vi "Copy Channel Properties.vi"(6 "Base Channel":string, 8 "error in (no error)":errorcluster, 9 "New Channel in":string, 10 "Group Name in":string, 11 "TDMS Log File in":refnum<class "TDMS Log File.lvclass">) -> (0 "error out":errorcluster, 1 "New Channel out":string, 2 "Group Name out":string, 3 "TDMS Log File out":refnum<class "TDMS Log File.lvclass">)   [LabVIEW 2015, in "TDMS Log File.lvclass"]
uses:
  TDMS Log File.lvclass
  TDMS Log File.lvclass/TDMS Log File.ctl
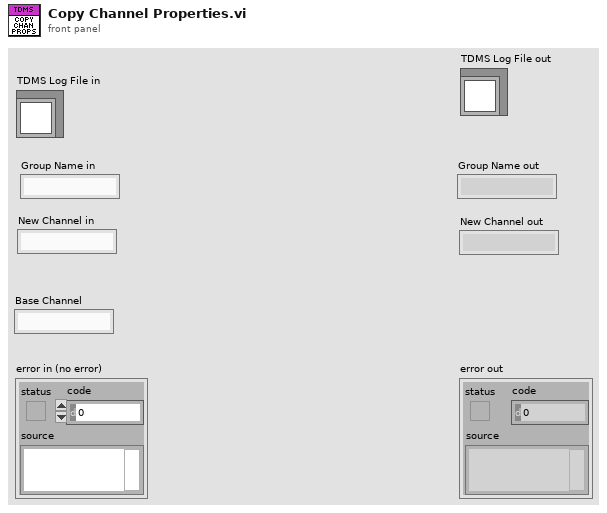
[diagram p1: front panel]
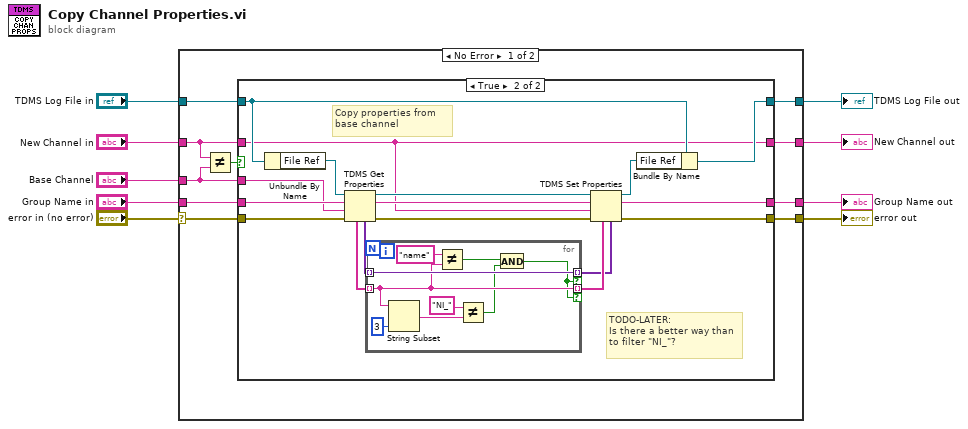
[diagram p0: block diagram]
diagram:
  n1 = case shown="No Error" "error in (no error)" {
    selector: "error in (no error)" -> [w11 w53]
    tunnel: [w10 w53] -> w8
    tunnel: [w12 w52] -> w6
    tunnel: "TDMS Log File in" -> [w13 w52]
    tunnel: "New Channel in" -> [w16 w50]
    tunnel: "Base Channel" -> [w17 _]
    tunnel: "Group Name in" -> [w18 w51]
    tunnel: [w15 w51] -> w2
    tunnel: [w14 w50] -> w1
    frame No Error {
      n2 = Not Equal?(x=w16, y=w17) -> (x != y?=w19:bool)
      n3 = case shown="True" w19 {
        tunnel: w18 -> [w22 w37]
        tunnel: w17 -> [_ w36]
        tunnel: w16 -> [w23 w28]
        tunnel: [w22 w35] -> w15
        tunnel: [w23 w28] -> w14
        tunnel: w13 -> [w21 w32]
        tunnel: [w21 w31] -> w12
        tunnel: w11 -> [w20 w30]
        tunnel: [w20 w29] -> w10
        frame False {
          # "Same channel name"
        }
        frame True {
          # "TODO-LATER:\nIs there a better way than\nto filter \"NI_\"?"
          # "Copy properties from \nbase channel"
          n4 = Unbundle By Name(w32) -> ("File Ref"=w34:refnum<k34>)
          n5 = TDMS Get Properties(8:w30, 9:w36, 10:w37, 11:w34) -> (0:w39:errorcluster, 2:w40:string, 3:w38:refnum<k34>, 4:w26:variant[], 6:w27:string[])  [unwired: 2 in, 1 out]
          n6 = for {
            tunnel: w27 -> [w44] mode=indexing
            tunnel: w26 -> [w49] mode=indexing
            tunnel: [w49] -> w24 mode=indexing if=w41
            tunnel: [w44] -> w25 mode=indexing if=w41
            n7 = String Subset(string=w44, length (rest)=3 ("length (rest)")) -> (substring=w47:string)  [unwired: 1 in]
            n8 = Not Equal?(x="name", y=w44) -> (x != y?=w45:bool)
            n9 = Not Equal?(x="NI_", y=w47) -> (x != y?=w42:bool)
            n10 = And(x=w45, y=w42) -> (x .and. y?=w41:bool)
          }
          n11 = TDMS Set Properties(5:w24, 7:w25, 8:w39, 9:w28, 10:w40, 11:w38) -> (0:w29:errorcluster, 2:w35:string, 3:w33:refnum<k34>)  [unwired: 1 out]
          n12 = Bundle By Name(cluster=w32, "File Ref"=w33) -> (w31:refnum<class "TDMS Log File.lvclass">)
        }
      }
    }
    frame Error {
    }
  }
  "error out" <- w8
  "TDMS Log File out" <- w6
  "New Channel out" <- w1
  "Group Name out" <- w2
